vi "WriteSetPoint Example.vi"() -> ()   [LabVIEW 2019]
uses:
  BrooksDLL.dll
panel:
  in  "SetPointCode":u16(ring) items=["in %", "in Selected Unit"]
  out "S2 String":string
  out "S1 String":string
  out "S2":u8 format="%.0x"
  out "S1":u8 format="%.0x"
  out "Function Output Comment":string
  in  "SetPoint":sgl format="%.2f"
  out "output param":i32
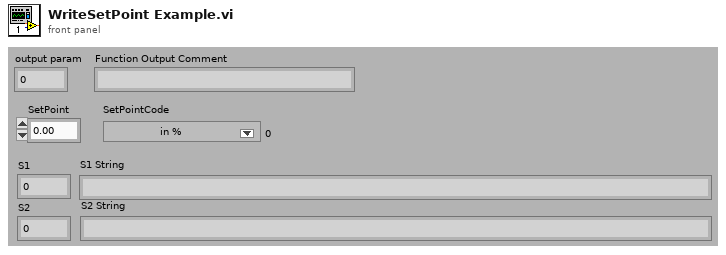
[diagram p1: front panel]
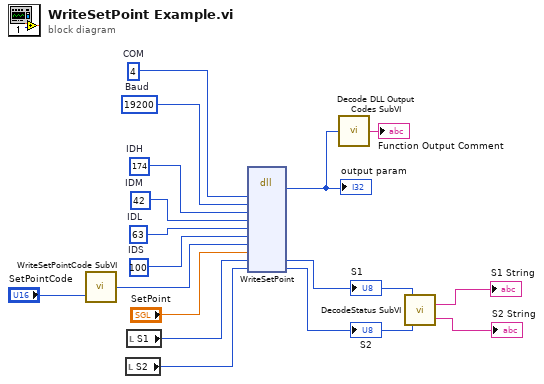
[diagram p0: block diagram]
diagram:
  w12 = u8 100  # IDS
  w13 = u8 63  # IDL
  w14 = u8 42  # IDM
  w15 = u8 174  # IDH
  w16 = 19200  # Baud
  w17 = 4  # COM
  n1 = call "WriteSetPointCode SubVI.vi"("SetPointCode 2"="SetPointCode") -> ("SetPointCode"=w2:u8)
  n2 = local read "S2"() -> (w5:u8)
  n3 = local read "S1"() -> (w4:u8)
  n4 = dll-call lib="G:/Developpement_de_Programmes/Programmes/Controle de pression/164J027_AD/Brooks DLL 1.0.1.0 32bit/Brooks DLL 1.0.1.0 Release 10032016/S Protocol/BrooksDLL.dll" fn="WriteSetPoint"("COM"=w17, "Baud"=w16, "IDH"=w15, "IDM"=w14, "IDL"=w13, "IDS"=w12, "SetPointCode"=w2, "SetPoint"="SetPoint", "S1"=w4, "S2"=w5) -> ("return type"=w11:i32, "S1"=w6:u8, "S2"=w7:u8)  [unwired: 11 in, 2 out]
  "output param" <- w11
  "S1" <- w6
  "S2" <- w7
  n5 = call "Decode DLL Output Codes SubVI.vi"("Numeric"=w11) -> ("Function Output Comment"=→"Function Output Comment":string)
  n6 = call "DecodeStatus SubVI.vi"("S2"=w7, "S1"=w6) -> ("S2 String"=→"S2 String":string, "S1 String"=→"S1 String":string)
